vi "TM_datasocket6.vi"() -> ()   [LabVIEW 2018]
panel:
  out "水平进度条":dbl(slide) scale=0.0..100.0
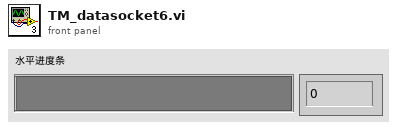
[diagram p1: front panel]
types:
  T1 = enum16{"Read", "Write", "ReadWrite", "BufferedRead", "BufferedReadWrite"}
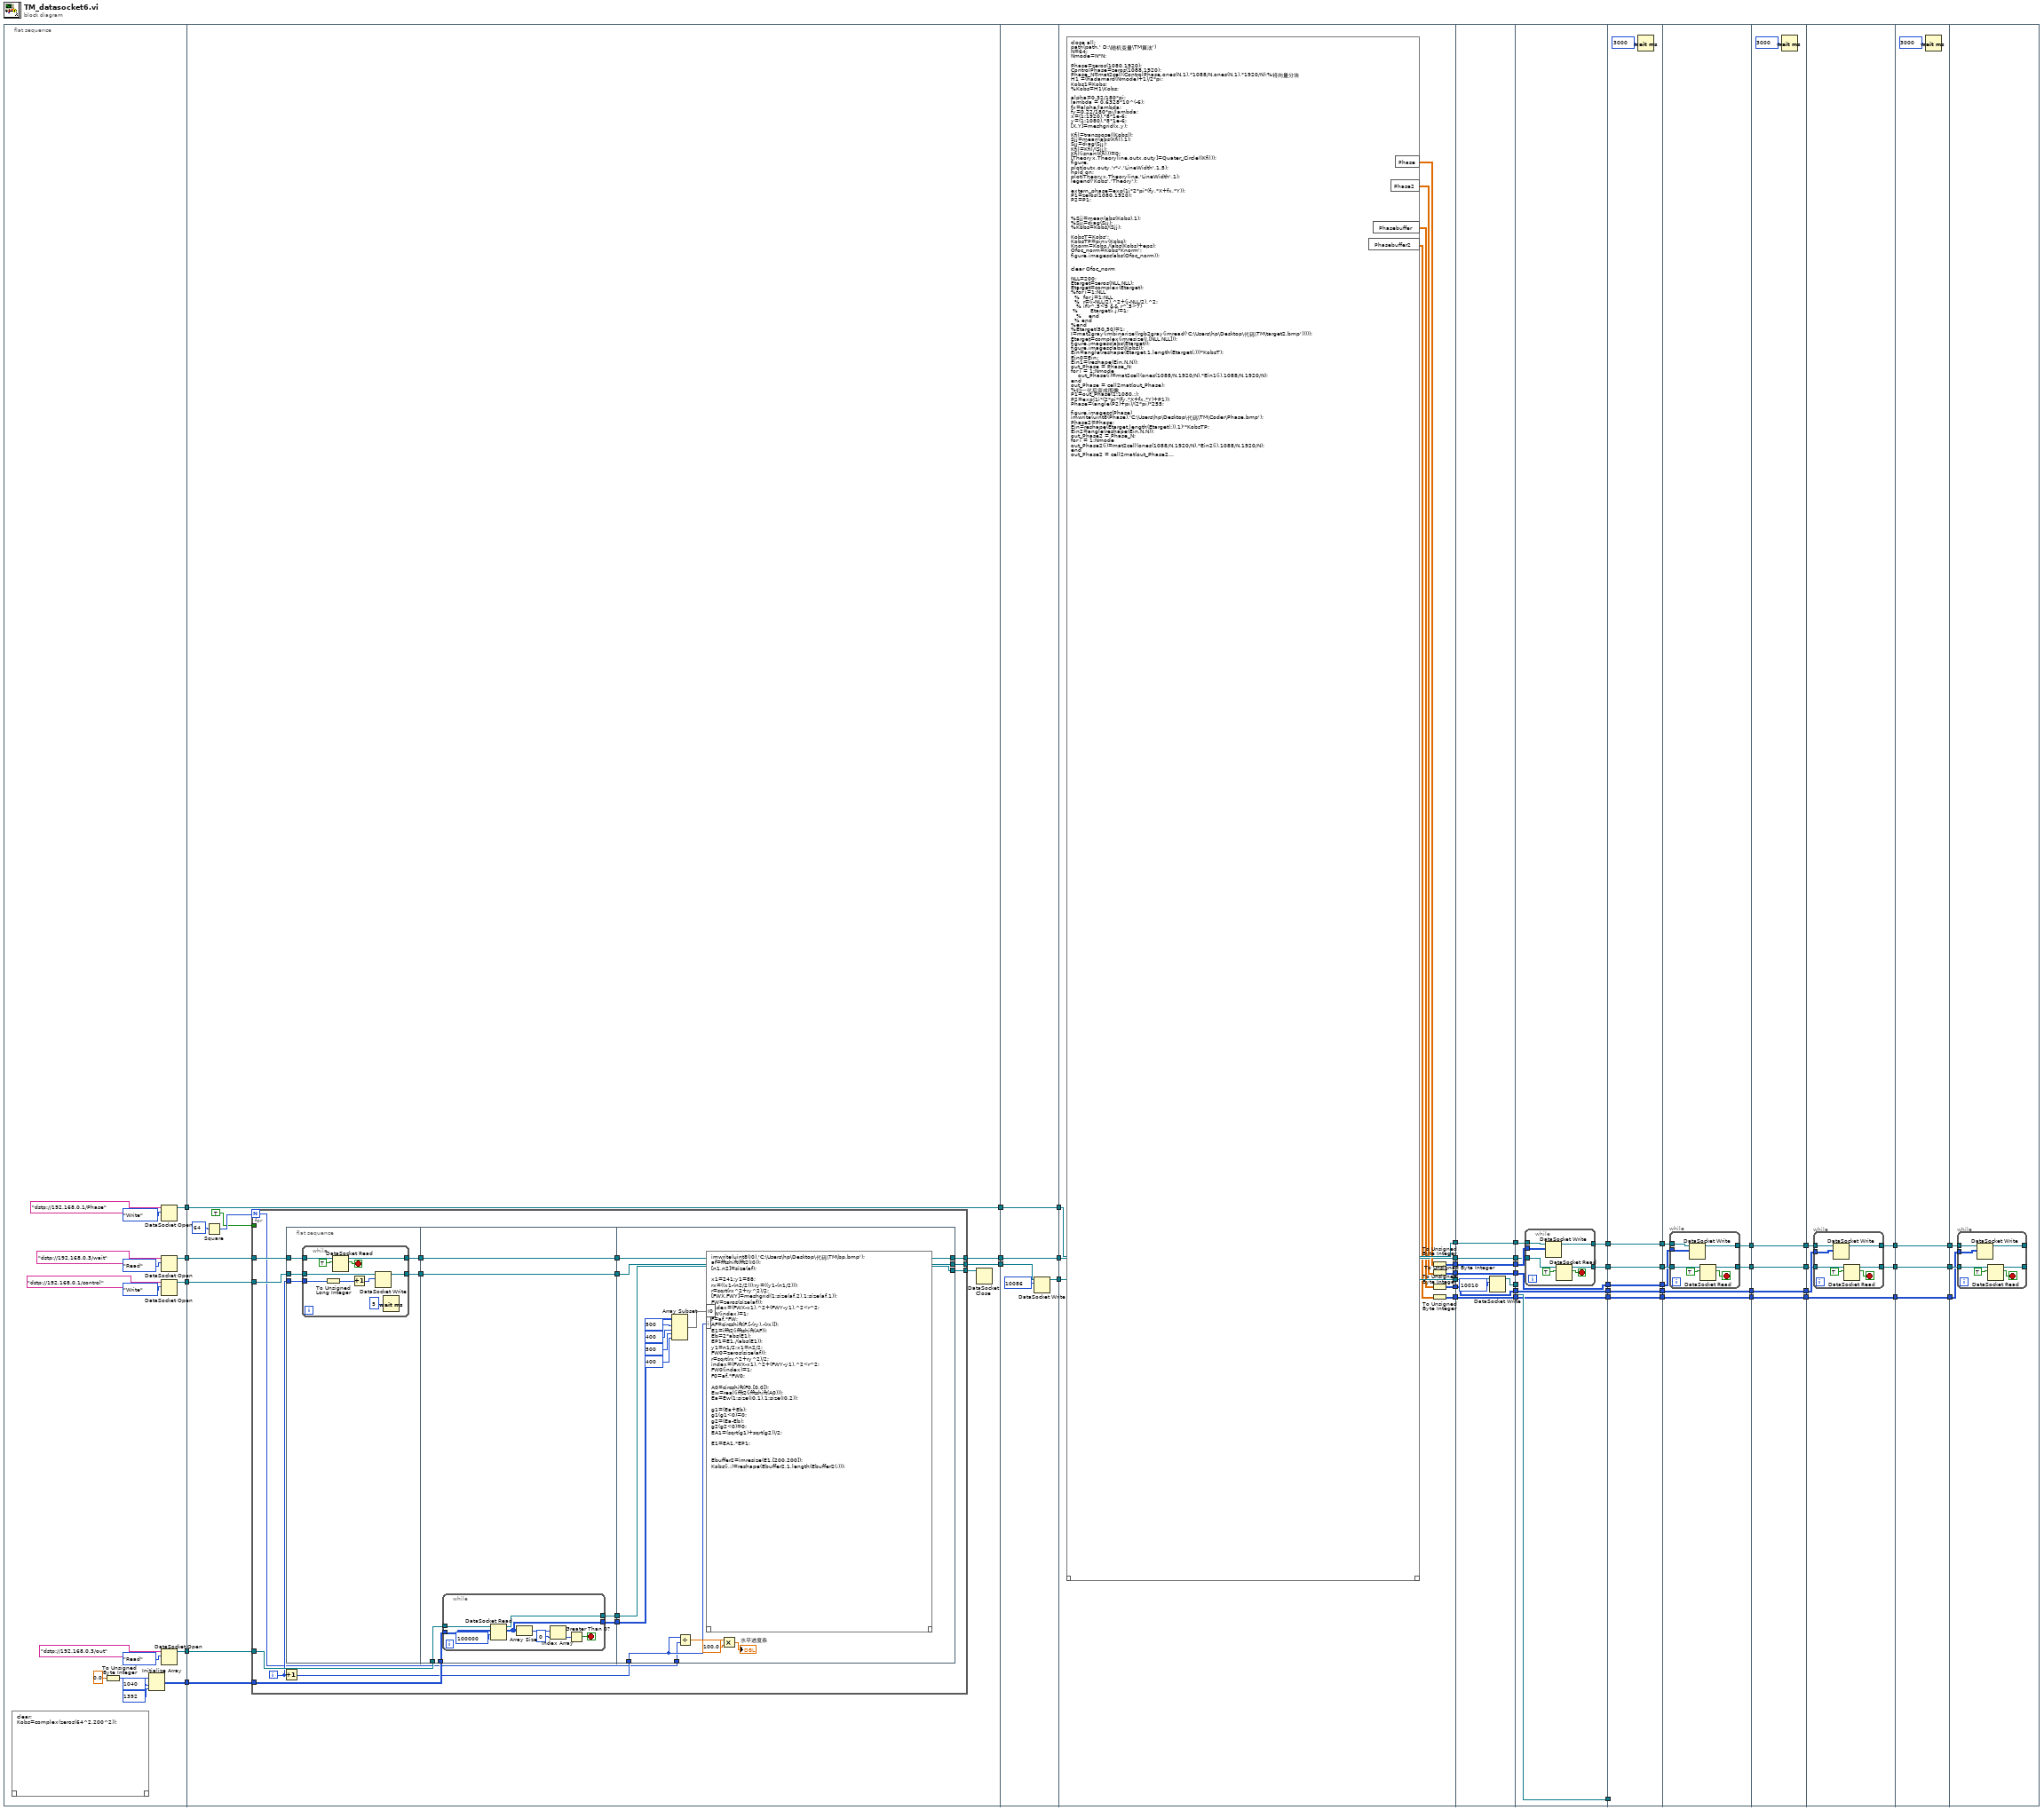
[diagram p0: block diagram]
diagram:
  n1 = flat-sequence {
    tunnel: [w63] -> w50
    tunnel: [w62] -> w49
    tunnel: [w59] -> w48
    tunnel: [w55] -> w47
    tunnel: [w56] -> w46
    tunnel: w50 -> [w76]
    tunnel: w49 -> [w75]
    tunnel: w48 -> [w71]
    tunnel: w47 -> [w74]
    tunnel: [w70] -> w45
    tunnel: w46 -> [w70]
    tunnel: [w69] -> w43
    tunnel: [w68] -> w35
    tunnel: w45 -> [w143]
    tunnel: [w143] -> w44
    tunnel: w43 -> [w142]
    tunnel: [w140] -> w37
    tunnel: [w139] -> w36
    tunnel: w35 -> [w139]
    tunnel: w44 -> [w154]
    tunnel: [w154] -> w42
    tunnel: [w152] -> w40
    tunnel: [w151] -> w38
    tunnel: w37 -> [w151]
    tunnel: w36 -> [w150]
    tunnel: [w150] -> w33
    tunnel: [w148] -> w26
    tunnel: [w146] -> w19
    tunnel: [w144] -> w1
    tunnel: w42 -> [w163]
    tunnel: [w163] -> w41
    tunnel: w40 -> [w162]
    tunnel: [w162] -> w39
    tunnel: w38 -> [w160]
    tunnel: [w159] -> w34
    tunnel: w33 -> [w159]
    tunnel: [w158] -> w31
    tunnel: w26 -> [w157]
    tunnel: [w157] -> w25
    tunnel: [w156] -> w20
    tunnel: w19 -> [w156]
    tunnel: [w155] -> w2
    tunnel: w1 -> [w155]
    tunnel: w41 -> [w171]
    tunnel: w39 -> [w172]
    tunnel: w34 -> [w170]
    tunnel: [w169] -> w32
    tunnel: w31 -> [w169]
    tunnel: [w168] -> w30
    tunnel: [w167] -> w27
    tunnel: w25 -> [w166]
    tunnel: [w166] -> w24
    tunnel: [w165] -> w21
    tunnel: w20 -> [w165]
    tunnel: [w164] -> w3
    tunnel: w2 -> [w164]
    tunnel: w32 -> [_]
    tunnel: w30 -> [w184]
    tunnel: [w184] -> w29
    tunnel: [w183] -> w28
    tunnel: w27 -> [w183]
    tunnel: w24 -> [w182]
    tunnel: [w182] -> w23
    tunnel: [w181] -> w22
    tunnel: w21 -> [w181]
    tunnel: [w180] -> w4
    tunnel: w3 -> [w180]
    tunnel: w29 -> [w192]
    tunnel: w28 -> [w191]
    tunnel: w23 -> [w190]
    tunnel: w22 -> [w189]
    tunnel: [w189] -> w18
    tunnel: [w188] -> w16
    tunnel: [w187] -> w14
    tunnel: [w186] -> w5
    tunnel: w4 -> [w186]
    tunnel: w18 -> [w204]
    tunnel: [w204] -> w17
    tunnel: w16 -> [w202]
    tunnel: [w202] -> w15
    tunnel: w14 -> [w201]
    tunnel: [w201] -> w13
    tunnel: [w200] -> w6
    tunnel: w5 -> [w200]
    tunnel: w17 -> [w210]
    tunnel: w15 -> [w209]
    tunnel: w13 -> [w208]
    tunnel: [w207] -> w12
    tunnel: [w206] -> w10
    tunnel: [w205] -> w7
    tunnel: w6 -> [w205]
    tunnel: w12 -> [w220]
    tunnel: [w220] -> w11
    tunnel: w10 -> [w219]
    tunnel: [w219] -> w9
    tunnel: [w218] -> w8
    tunnel: w7 -> [w218]
    tunnel: w11 -> [w224]
    tunnel: w9 -> [w223]
    tunnel: w8 -> [w222]
    frame #0 {
      n2 = script code="clear;\nKobs=complex(zeros(64^2,200^2));"() -> ()  [unwired: 1 in, 1 out]
      n3 = To Unsigned Byte Integer(number=0.0 ("元素")) -> (unsigned 8bit integer=w51:u8)
      n4 = Initialize Array(w51, 1040 ("维数大小"), 1392 ("维数大小")) -> (w55:u8[][])
      n5 = DataSocket Open(10:T1."Write" ("模式"), 11:"dstp://192.168.0.1/Phase" ("URL")) -> (3:w56:refnum<k13>)  [unwired: 2 in, 1 out]
      n6 = DataSocket Open(10:T1."Read" ("模式"), 11:"dstp://192.168.0.3/wait" ("URL")) -> (3:w59:refnum<k13>)  [unwired: 2 in, 1 out]
      n7 = DataSocket Open(10:T1."Write" ("模式"), 11:"dstp://192.168.0.1/control" ("URL")) -> (3:w63:refnum<k13>)  [unwired: 2 in, 1 out]
      n8 = DataSocket Open(10:T1."Read" ("模式"), 11:"dstp://192.168.0.3/out" ("URL")) -> (3:w62:refnum<k13>)  [unwired: 2 in, 1 out]
    }
    frame #1 {
      n9 = Square(x=64) -> (x^2=w77:i32)
      n10 = for {
        N: w77 -> [w79]
        tunnel: w76 -> [w81]
        tunnel: [w94] -> w69
        tunnel: w75 -> [w93]
        tunnel: w74 -> [w92]
        tunnel: [w91] -> w73
        tunnel: TRUE -> [_]
        tunnel: w71 -> [w86]
        tunnel: [w83] -> w68
        i -> [w82]
        n11 = Increment(x=w82) -> (x+1=w80:i32)
        n12 = flat-sequence {
          tunnel: [w95] -> w87
          tunnel: [w98] -> w84
          tunnel: w82 -> [w97]
          tunnel: w81 -> [w96]
          tunnel: w86 -> [w99]
          tunnel: w87 -> [w115]
          tunnel: w93 -> [w114]
          tunnel: w92 -> [w113]
          tunnel: [w115] -> w90
          tunnel: [w112] -> w89
          tunnel: [w111] -> w88
          tunnel: [w110] -> w85
          tunnel: w84 -> [w110]
          tunnel: [w137] -> w91
          tunnel: [w138] -> w94
          tunnel: w90 -> [w138]
          tunnel: w89 -> [w137]
          tunnel: w88 -> [w130]
          tunnel: w80 -> [w135]
          tunnel: [w136] -> w83
          tunnel: w85 -> [w136]
          tunnel: w79 -> [w134]
          frame #0 {
            n13 = while {
              tunnel: w99 -> [w109]
              tunnel: [w106] -> w98
              tunnel: w97 -> [w103]
              tunnel: w96 -> [w102]
              tunnel: [w101] -> w95
              stop <- w107 stop-if-true
              n14 = To Unsigned Long Integer(number=w103) -> (unsigned 32bit integer=w105:u32)
              n15 = DataSocket Read(10:TRUE, 11:w109) -> (2:w107:bool, 3:w106:refnum<k13>)  [unwired: 3 in, 5 out]
              n16 = Increment(x=w105) -> (x+1=w104:u32)
              n17 = DataSocket Write(10:w104, 11:w102) -> (3:w101:refnum<k13>)  [unwired: 2 in, 2 out]
              n18 = Wait (ms)(milliseconds to wait=u32 5 ("等待时间（毫秒）")) -> ()  [unwired: 1 out]
            }
          }
          frame #1 {
            n19 = while {
              tunnel: w114 -> [w124]
              tunnel: [w122] -> w112
              tunnel: w113 -> [w123]
              tunnel: [w120] -> w111
              stop <- w119 stop-if-true
              n20 = DataSocket Read(9:100000 ("毫秒超时(10000)"), 10:w123, 11:w124) -> (2:w120:u8[][], 3:w122:refnum<k13>)  [unwired: 2 in, 5 out]
              n21 = Array Size(array=w120) -> (size(s)=w118:i32[])
              n22 = Index Array(array=w118, index=0 ("索引")) -> (element=w116:i32)
              n23 = Greater Than 0?(x=w116) -> (x > 0?=w119:bool)
            }
          }
          frame #2 {
            n24 = Array Subset(array=w130, index (row)=500 ("索引"), length (row)=400 ("长度"), index (col)=500 ("索引"), length (col)=400 ("长度")) -> (w125:u8[][])
            n25 = Divide(x=w135, y=w134) -> (x/y=w133:dbl)
            n26 = script code="imwrite(uint8(I0),'C:\\Users\\hp\\Desktop\\代码\\TM\\bp.bmp');\naf=fftshift(fft2(I0));\n[n1,n2]=size(af);\n\nx1=241;y1=88;\nrx=((x1-(n2/2)));ry=((y1-(n1/2)));\nr=sqrt(rx^2+ry^2)/2;\n[FWX,FWY]=meshgrid(1:size(af,2),1:size(af,1));\nFW=zeros(size(af));\nindex=(FWX-x1).^2+(FWY-y1).^2<r^2;\nFW(index)=1;\nF=af.*FW;\nAF=circshift(F,[-(ry),-(rx)]);\nE1=ifft2(ifftshift(AF));\nEb=2*abs(E1);\nEP1=E1./(abs(E1));\ny1=n1/2;x1=n2/2;\nFW0=zeros(size(af));\nr=sqrt(rx^2+ry^2)/2;\nindex=(FWX-x1).^2+(FWY-y1).^2<r^2;\nFW0(index)=1;\nF0=af.*FW0;\n\nA0=circshift(F0,[0,0]);\nEw=real(ifft2(ifftshift(A0)));\nEa=Ew(1:size(I0,1),1:size(I0,2));\n\ng1=(Ea+Eb);\ng1(g1<0)=0;\ng2=(Ea-Eb);\ng2(g2<0)=0;\nEA1=(sqrt(g1)+sqrt(g2))/2;\n\nE1=EA1.*EP1;\n\n\nEbuffer2=imresize(E1,[200,200]);\nKobs(i,:)=reshape(Ebuffer2,1,length(Ebuffer2(:)));"("I0"=w125, "i"=w135) -> ()  [unwired: 1 in, 1 out]
            n27 = Multiply(x=w133, y=100.0) -> (x*y=→"水平进度条":dbl)
          }
        }
      }
      n28 = DataSocket Close(11:w73) -> ()  [unwired: 2 in, 2 out]
    }
    frame #2 {
      n29 = DataSocket Write(10:10086, 11:w142) -> (3:w140:refnum<k13>)  [unwired: 2 in, 2 out]
    }
    frame #3 {
      n30 = script code="close all;\npath(path,' D:\\随机变量\\TM算法')\nN=64;\nNmode=N*N;\n\nPhase=zeros(1080,1920);\nControlPhase=zeros(1088,1920);\nPhase_N=mat2cell(ControlPhase,ones(N,1).*1088/N,ones(N,1).*1920/N);%将向量分块\nH1 =(hadamard(Nmode)+1)/2*pi; \nKobs1=Kobs;\n%Kobs=H1\\Kobs;\n\nalpha=0.32/180*pi;\nlambda = 0.6328*10^(-6);\nfx=alpha/lambda;\nfy=0.22/180*pi/lambda;\nx=(1:1920).*8*1e-6;\ny=(1:1080).*8*1e-6;\n[X,Y]=meshgrid(x,y);\n\nKfil=transpose((Kobs));\nSjj=mean(abs(Kfil),1); \nSjj=diag(Sjj);\nKfil=Kfil/(Sjj);\nKfil(isnan(Kfil))=0;\n[Theoryx,Theoryline,outx,outy]=Quater_Circle((Kfil));\nfigure,\nplot(outx,outy,'r*-','LineWidth',1.5);\nhold on;\nplot(Theoryx,Theoryline,'LineWidth',1);\nlegend('Kobs','Theory');\n\nextern_phase=exp(1i*2*pi*(fy.*X+fx.*Y));\nP1=zeros(1080,1920);\nP2=P1;\n\n\n\n%Sjj=mean(abs(Kobs),1);\n%Sjj=diag(Sjj);\n%Kobs=Kobs/(Sjj);\n\nKobsT=Kobs';\nKobsTP=pinv(Kobs);\nKnorm=Kobs./(abs(Kobs)+eps);\nOfoc_norm=Kobs*Knorm';\nfigure,imagesc(abs(Ofoc_norm));\n\n\nclear Ofoc_norm\n\nNLL=200;\nEtarget=zeros(NLL,NLL);\nEtarget=complex(Etarget);\n%for i=1:NLL\n  %  for j=1:NLL\n  %  r=(i-NLL/2).^2+(j-NLL/2).^2;\n   % if(r^.5<9 && r^.5>7)\n %       Etarget(i,j)=1;\n   %    end\n  % end\n%end\n%Etarget(50,50)=1;\nI=mat2gray(imbinarize((rgb2gray(imread('C:\\Users\\hp\\Desktop\\代码\\TM\\target2.bmp')))));\nEtarget=complex(imresize(I,[NLL,NLL]));\nfigure,imagesc(abs(Etarget));\nfigure,imagesc(abs(Kobs));\nEin=angle(reshape(Etarget,1,length(Etarget(:)))*KobsT);\nEin0=Ein;\nEin1=(reshape(Ein,N,N));\nout_Phase = Phase_N;\nfor i = 1:Nmode\n    out_Phase(i)=mat2cell(ones(1088/N,1920/N).*Ein1(i),1088/N,1920/N);\nend\nout_Phase = cell2mat(out_Phase);\n%归一化后变成图像\nP1=out_Phase(1:1080,:);\nP2=exp(1i*(2*pi*(fy.*X+fx.*Y)+P1));\nPhase=(angle(P2)+pi)/(2*pi)*255;\n\nfigure,imagesc(Phase)\nimwrite(uint8(Phase),'C:\\Users\\hp\\Desktop\\代码\\TM\\Coder\\Phase.bmp');\nPhase2=Phase; \nEin=reshape(Etarget,length(Etarget(:)),1)'*KobsTP;\nEin2=angle(reshape(Ein,N,N));\nout_Phase2 = Phase_N;\nfor i = 1:Nmode\nout_Phase2(i)=mat2cell(ones(1088/N,1920/N).*Ein2(i),1088/N,1920/N);\nend\nout_Phase2 = cell2mat(out_Phase2);\nP1=out_Phase2(1:1080,:);\nP2=exp(1i*(2*pi*(fy.*X+fx.*Y)+P1));\nPhase2=(angle(P2)+pi)/(2*pi)*255;\nfigure,imagesc(Phase2)\nimwrite(uint8(Phase2),'C:\\Users\\hp\\Desktop\\代码\\TM\\Coder\\Phase2.bmp');\n\ninter=100;\nU0=ones(size(Phase2)).*exp(1i*Phase2);\nPhasebuffer=Phase2;\nUinverse_phase=exp(1i*(angle(Ein)+pi));\nEtarget1=reshape(Etarget,length(Etarget(:)),1);\nfor k=1:inter \n    Uout=(ones(length(Uinverse_phase),1)'*255).*Uinverse_phase*Kobs;\n    Uinverse_in=exp(1i*angle(Uout)).*abs(Etarget1)';\n    Uinverse_out=Uinverse_in*KobsTP;\n    Uinverse_phase=Uinverse_out./abs(Uinverse_out);\nend\nUout=reshape(Uout,NLL,NLL);\nfigure,imagesc(abs(Uout));\nUinverse_phase=angle(Uinverse_phase);\nout_Phasebuffer = Phase_N;\n    for i = 1:Nmode\n      out_Phasebuffer(i)=mat2cell(ones(1088/N,1920/N).*Uinverse_phase(i),1088/N,1920/N);\n    end\nout_Phasebuffer = cell2mat(out_Phasebuffer);\nP1=out_Phasebuffer(1:1080,:);\nP2=exp(1i*(2*pi*(fy.*X+fx.*Y)+P1));\nPhasebuffer=(angle(P2)+pi)/(2*pi)*255;\nfigure,imagesc(Phasebuffer)\nimwrite(uint8(Phasebuffer),'C:\\Users\\hp\\Desktop\\代码\\TM\\Coder\\Phasebuffer2000.bmp');\nalpha=0.32/180*pi;\nlambda = 0.6328*10^(-6);\nfx=alpha/lambda;\nfy=0.22/180*pi/lambda;\nx=(1:1920).*8*1e-6;\ny=(1:1080).*8*1e-6;\n[X,Y]=meshgrid(x,y);\n[Aout,~]=GA_P(transpose(Kobs),angle(Ein)+pi,Etarget1,50,N);\nout_Phasebuffer2= Phase_N;\nfor i = 1:Nmode\n      out_Phasebuffer2(i)=mat2cell(ones(1088/N,1920/N).*Aout(i),1088/N,1920/N);\n end\nout_Phasebuffer2 = cell2mat(out_Phasebuffer2);\nP1=out_Phasebuffer2(1:1080,:);\nP2=exp(1i*(2*pi*(fy.*X+fx.*Y)+P1));\nPhasebuffer2=(angle(P2)+pi)/(2*pi)*255;\nfigure,imagesc(Phasebuffer2)\nimwrite(uint8(Phasebuffer2),'C:\\Users\\hp\\Desktop\\代码\\TM\\Coder\\Phasebuffer22000.bmp');"() -> ("Phase"=w153:dbl[][], "Phase2"=w149:dbl[][], "Phasebuffer"=w147:dbl[][], "Phasebuffer2"=w145:dbl[][])  [unwired: 1 in, 1 out]
      n31 = To Unsigned Byte Integer(number=w153) -> (unsigned 8bit integer=w152:u8[][])
      n32 = To Unsigned Byte Integer(number=w149) -> (unsigned 8bit integer=w148:u8[][])
      n33 = To Unsigned Byte Integer(number=w147) -> (unsigned 8bit integer=w146:u8[][])
      n34 = To Unsigned Byte Integer(number=w145) -> (unsigned 8bit integer=w144:u8[][])
    }
    frame #4 {
      n35 = DataSocket Write(10:10010, 11:w160) -> (3:w158:refnum<k13>)  [unwired: 2 in, 2 out]
    }
    frame #5 {
      n36 = while {
        tunnel: w172 -> [w179]
        tunnel: w170 -> [w176]
        tunnel: [w173] -> w167
        tunnel: w171 -> [w177]
        tunnel: [w178] -> w168
        stop <- w174 stop-if-true
        n37 = DataSocket Write(10:w179, 11:w177) -> (3:w178:refnum<k13>)  [unwired: 2 in, 2 out]
        n38 = DataSocket Read(10:TRUE, 11:w176) -> (2:w174:bool, 3:w173:refnum<k13>)  [unwired: 3 in, 5 out]
      }
    }
    frame #6 {
      n39 = Wait (ms)(milliseconds to wait=u32 3000 ("等待时间（毫秒）")) -> ()  [unwired: 1 out]
    }
    frame #7 {
      n40 = while {
        tunnel: w190 -> [w199]
        tunnel: w191 -> [w196]
        tunnel: [w193] -> w187
        tunnel: w192 -> [w197]
        tunnel: [w198] -> w188
        stop <- w194 stop-if-true
        n41 = DataSocket Write(10:w199, 11:w197) -> (3:w198:refnum<k13>)  [unwired: 2 in, 2 out]
        n42 = DataSocket Read(10:TRUE, 11:w196) -> (2:w194:bool, 3:w193:refnum<k13>)  [unwired: 3 in, 5 out]
      }
    }
    frame #8 {
      n43 = Wait (ms)(milliseconds to wait=u32 3000 ("等待时间（毫秒）")) -> ()  [unwired: 1 out]
    }
    frame #9 {
      n44 = while {
        tunnel: w210 -> [w217]
        tunnel: w208 -> [w214]
        tunnel: [w211] -> w206
        tunnel: w209 -> [w215]
        tunnel: [w216] -> w207
        stop <- w212 stop-if-true
        n45 = DataSocket Write(10:w217, 11:w215) -> (3:w216:refnum<k13>)  [unwired: 2 in, 2 out]
        n46 = DataSocket Read(10:TRUE, 11:w214) -> (2:w212:bool, 3:w211:refnum<k13>)  [unwired: 3 in, 5 out]
      }
    }
    frame #10 {
      n47 = Wait (ms)(milliseconds to wait=u32 3000 ("等待时间（毫秒）")) -> ()  [unwired: 1 out]
    }
    frame #11 {
      n48 = while {
        tunnel: w222 -> [w231]
        tunnel: w223 -> [w228]
        tunnel: [w225] -> _
        tunnel: w224 -> [w229]
        tunnel: [w230] -> _
        stop <- w226 stop-if-true
        n49 = DataSocket Write(10:w231, 11:w229) -> (3:w230:refnum<k13>)  [unwired: 2 in, 2 out]
        n50 = DataSocket Read(10:TRUE, 11:w228) -> (2:w226:bool, 3:w225:refnum<k13>)  [unwired: 3 in, 5 out]
      }
    }
  }
